vi "XY Graph Sliced Mean, SDV & CV Plots Event.vi"(8 "Error In":errorcluster, 10 "Mouse Coordinates":T1, 11 "Multiplot XY Graph":T2) -> (0 "Error Out":errorcluster, 1 "Message":string)   [LabVIEW 2021, in "XY Graph Add-Ons.lvlib"]
uses:
  XY Graph Add-Ons.lvlib
  XY Graph Refnum.ctl
  <vilib>/Utility/miscctls.llb/LVPoint32TypeDef.ctl
  Get Plot at Mouse Click (XY Graph)/Get Plot at Mouse Click [AAC].vi
  XY Graph Add Multiplots with Names.vi
  Graphs.lvlib
  Variant/Variant.lvlib
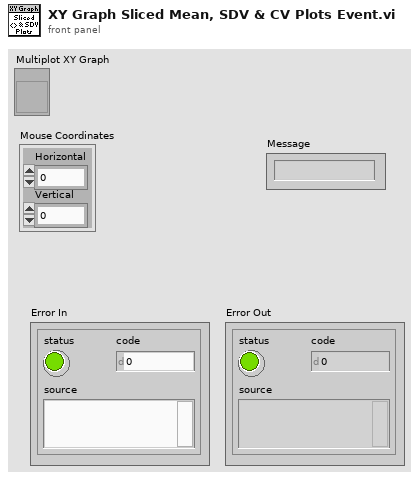
[diagram p1: front panel]
types:
  T1 = typedef "LVPoint32TypeDef.ctl" = cluster{"Horizontal":i32, "Vertical":i32}
  T2 = typedef "XY Graph Add-Ons.lvlib/XY Graph Refnum.ctl" = refnum<vi>
  T3 = typedef "XY Graph Add-Ons.lvlib/XY Graph Sliced Mean & SDV Step Definition.ctl" = cluster{"Axis Start":dbl, "Axis Stop":dbl, "# Steps":i32, "Step Size":dbl, "Step Definition":enum32{"# Steps", "Step Size"}, "Upper Percentile":dbl, "Lower Percentile":dbl, "Min # Data Points/Slice":i32, "Output Abscissa Statistics Plots":bool, "Bin Location":T4}
  T4 = typedef "XY Graph Add-Ons.lvlib/XY Graph Sliced CV Abscissa Location.ctl" = enum16{"Left", "Center", "Mean", "Right"}
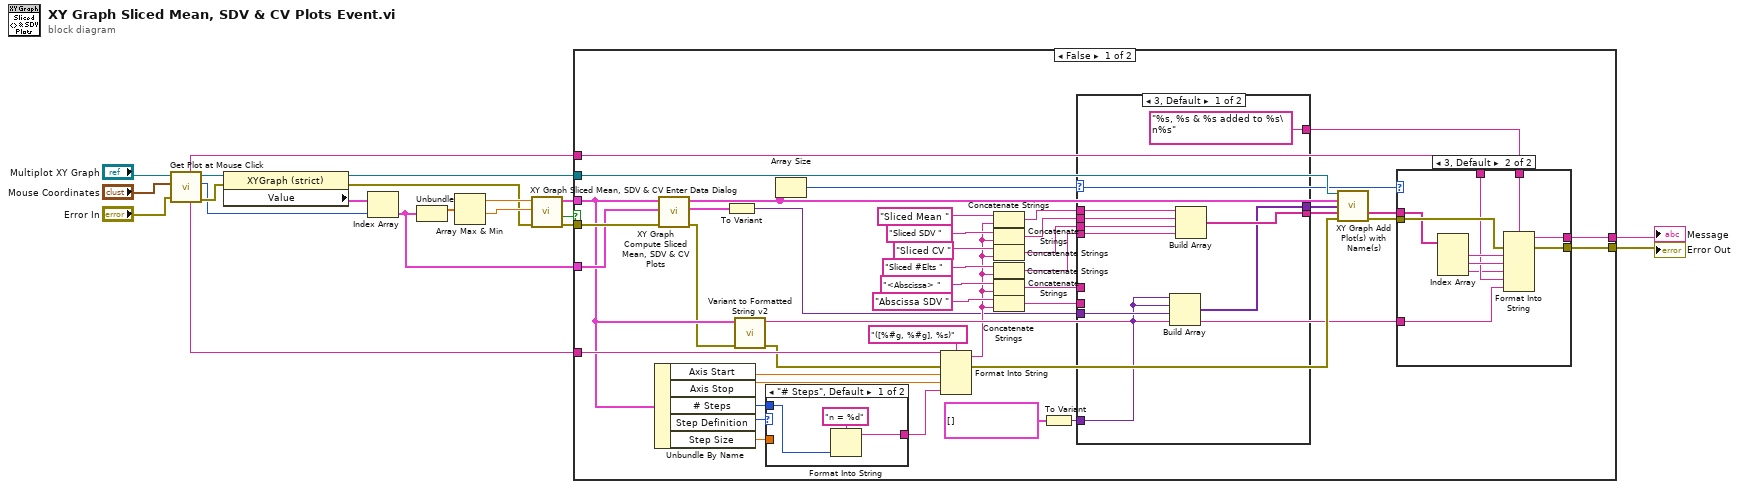
[diagram p0: block diagram]
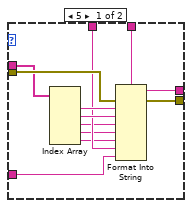
[diagram p2: hidden frame]
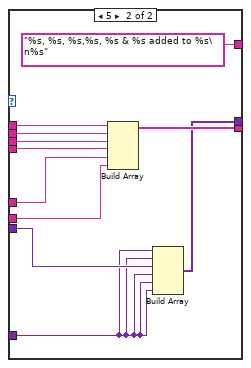
[diagram p3: hidden frame]
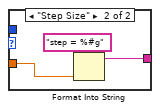
[diagram p4: hidden frame]
diagram:
  n1 = call-poly "Get Plot at Mouse Click.vi"("error in (no error)"="Error In", "Mouse Click Coordinates"="Mouse Coordinates", "XYGraph Ref"="Multiplot XY Graph") -> ("error out"=w18:errorcluster, "Plot at Coordinates"=w16:i32, "XYGraph Ref"=w19:T2, "Plot Name"=w4:string, "Graph Name"=w14:string)  [unwired: 2 in, 2 out]
  n2 = property class="XYGraph (strict)"(reference=w19, error in=w18) -> (reference out=w15:T2, error out=w8:errorcluster, "Value"=w17:cluster{"X Array":dbl[], "Y Array":dbl[]}[])
  n3 = Index Array(array=w17, index=w16) -> (element=w6:cluster{"X Array":dbl[], "Y Array":dbl[]})
  n4 = Unbundle(w6) -> ("X Array"=w11:dbl[])  [unwired: 1 out]
  n5 = Array Max & Min(array=w11) -> (max value=w10:dbl, min value=w9:dbl)  [unwired: 2 out]
  n6 = call "XY Graph Sliced Mean, SDV & CV Enter Data Dialog.vi"("Error In"=w8, "X min"=w9, "X max"=w10) -> ("Error Out"=w7:errorcluster, "Cancelled?"=w1:bool, "Slices Definition"=w5:T3)  [unwired: 6 in]
  n7 = case shown="False" w1 {
    tunnel: w15 -> [w63 _]
    tunnel: w14 -> [w50 _]
    tunnel: [w61 _] -> w13
    tunnel: [w60 w112] -> w12
    tunnel: w7 -> [w59 w112]
    tunnel: w6 -> [w58 _]
    tunnel: w5 -> [w39 _]
    tunnel: w4 -> [w57 _]
    frame False {
      n8 = Unbundle By Name(w39) -> ("Axis Start"=w49:dbl, "Axis Stop"=w48:dbl, "# Steps"=w52:i32, "Step Definition"=w53:enum32{"# Steps", "Step Size"}, "Step Size"=w51:dbl)
      n9 = call "XY Graph Compute Sliced Mean, SDV & CV Plots.vi"("error in (no error)"=w59, "Plot"=w58, "Slices Definition"=w39) -> ("error out"=w31:errorcluster, "Bin Intensity Distribution"=w25:cluster{"Intensity Array":sgl[]}[], "Plots"=w36:cluster{"X Array":dbl[], "Y Array":dbl[]}[])  [unwired: 6 in]
      n10 = To Variant(anything=w25) -> (Variant=w22:variant)
      n11 = call "Variant to Formatted String v2.vi"("error in (no error)"=w31, "Anything"=w39) -> ("error out"=w38:errorcluster, "String"=w37:string)  [unwired: 8 in]
      n12 = case shown="\"# Steps\", Default" w53 {
        tunnel: w52 -> [w108 _]
        tunnel: [w106 w110] -> w47
        tunnel: w51 -> [_ w109]
        frame "# Steps", Default {
          n13 = Format Into String(format string="n = %d", w108) -> (resulting string=w106:string)  [unwired: 2 in, 1 out]
        }
        frame "Step Size" {
          n14 = Format Into String(format string="step = %#g", w109) -> (resulting string=w110:string)  [unwired: 2 in, 1 out]
        }
      }
      n15 = Array Size(array=w36) -> (size(s)=w26:i32)
      n16 = Format Into String(format string="([%#g, %#g], %s)", initial string=w57, error in=w38, w49, w48, w47) -> (resulting string=w29:string, error out=w46:errorcluster)
      n17 = Concatenate Strings("Sliced Mean " ("format string"), w29) -> (w42:string)
      n18 = Concatenate Strings("Sliced SDV " ("format string"), w29) -> (w41:string)
      n19 = Concatenate Strings("Sliced CV " ("format string"), w29) -> (w28:string)
      n20 = Concatenate Strings("Sliced #Elts " ("format string"), w29) -> (w40:string)
      n21 = Concatenate Strings("<Abscissa> " ("format string"), w29) -> (w35:string)
      n22 = Concatenate Strings("Abscissa SDV " ("format string"), w29) -> (w34:string)
      n23 = To Variant(anything=cluster{"Intensity Array":sgl[]}[] [] ("Bin Intensity Distribution")) -> (Variant=w23:variant)
      n24 = case shown="3, Default" w26 {
        tunnel: [w94 w105] -> w55
        tunnel: w42 -> [w93 w104]
        tunnel: w41 -> [w92 w103]
        tunnel: w40 -> [w90 w102]
        tunnel: w35 -> [_ w101]
        tunnel: w34 -> [_ w100]
        tunnel: w28 -> [w91 w99]
        tunnel: ["%s, %s & %s added to %s\n%s" ("format string") "%s, %s, %s,%s, %s & %s added to %s\n%s" ("format string")] -> w27
        tunnel: w22 -> [w88 w97]
        tunnel: [w86 w96] -> w21
        tunnel: w23 -> [w87 w95]
        frame 3, Default {
          n25 = Build Array(w87, w87, w88, w87) -> (w86:variant[])
          n26 = Build Array(w93, w92, w91, w90) -> (w94:string[])
        }
        frame 5 {
          n27 = Build Array(w104, w103, w99, w102, w101, w100) -> (w105:string[])
          n28 = Build Array(w95, w95, w97, w95, w95, w95) -> (w96:variant[])
        }
      }
      n29 = call-poly "XY Graph Add Plot(s) with Name(s).vi"("XYGraph in"=w63, "Array of Plots"=w36, "Plots Metadata"=w21, "Array of Plot Names (\"Plot\")"=w55, "error in (no error)"=w46) -> ("Added Plot Names"=w54:string[], "error out"=w62:errorcluster)  [unwired: 6 in, 3 out]
      n30 = case shown="3, Default" w26 {
        tunnel: w62 -> [w75 w85]
        tunnel: [w74 w84] -> w61
        tunnel: [w73 w83] -> w60
        tunnel: w54 -> [w72 w82]
        tunnel: w50 -> [w69 w79]
        tunnel: w37 -> [w67 w77]
        tunnel: w27 -> [w66 w76]
        frame 5 {
          n31 = Index Array(array=w72) -> (element #1=w71:string, element #2=w70:string, element #3=w68:string, element #4=w65:string, element #5=w64:string)  [unwired: 5 in]
          n32 = Format Into String(format string=w66, error in=w75, w71, w70, w68, w65, w64, w69, w67) -> (resulting string=w74:string, error out=w73:errorcluster)  [unwired: 1 in]
        }
        frame 3, Default {
          n33 = Index Array(array=w82) -> (element #1=w81:string, element #2=w80:string, element #3=w78:string)  [unwired: 3 in]
          n34 = Format Into String(format string=w76, error in=w85, w81, w80, w78, w79, w77) -> (resulting string=w84:string, error out=w83:errorcluster)  [unwired: 1 in]
        }
      }
    }
    frame True {
      # "Cancelled"
    }
  }
  "Error Out" <- w12
  "Message" <- w13
